vi "TCU Settings Dialog.vi"(8 "error in (no error)":errorcluster, 10 "Message Queues":T11, 11 "TCU Module State Cluster In":T1={"TCU Module Config"={"GUID"="", "Drop Coords"={"Horizontal"=0, "Vertical"=0}, "Process Name"="", "Queue Name"="", "Settings"={"Cycle Period"=500.0, "Setpoint Entry"=0.0, "Output Device"=enum."Default", "Huber Ministat 230 Settings"={"VISA resource name"="", "Simulated?"=TRUE}, "Lauda Settings"={"VISA resource name"="", "Simulated?"=FALSE, "Pump Power"=2}, "Julabo FP-50 Settings"={"VISA resource name"="", "Simulated?"=FALSE, "Pump Power"=2}, "Internal Control?"=FALSE, "Huber Unistat 410 Settings"={"VISA resource name"="", "Address"=0, "Simulated?"=FALSE}}, "Load Count"=0, "Power Level Changed"=FALSE}, "State"=enum."Idle", "Start Time"=timestamp(0 s since 1904-01-01), "Current Time"=timestamp(0 s since 1904-01-01), "First Iteration"=FALSE, "Data"={"TCU Temp"=0.0}, "Process Name"="", "TCU On?"=FALSE, "Power Level Changed"=FALSE} {"TCU Module Config"."Settings"."Huber Unistat 410 Settings"."Address" min=0 max=99 format="%02.0f"; "TCU Module Config"."Settings"."Julabo FP-50 Settings"."Pump Power" min=0 max=8 step=1; "TCU Module Config"."Settings"."Lauda Settings"."Pump Power" min=0 max=8 step=1}) -> (0 "error out":errorcluster, 1 "Cancelled?":bool=TRUE, 2 "UI Refresh Needed?":bool, 3 "TCU Module Config Out":T2={"GUID"="", "Drop Coords"={"Horizontal"=0, "Vertical"=0}, "Process Name"="", "Queue Name"="", "Settings"={"Cycle Period"=0.0, "Setpoint Entry"=0.0, "Output Device"=enum."Default", "Huber Ministat 230 Settings"={"VISA resource name"="", "Simulated?"=FALSE}, "Lauda Settings"={"VISA resource name"="", "Simulated?"=FALSE, "Pump Power"=2}, "Julabo FP-50 Settings"={"VISA resource name"="", "Simulated?"=FALSE, "Pump Power"=2}, "Internal Control?"=FALSE, "Huber Unistat 410 Settings"={"VISA resource name"="", "Address"=0, "Simulated?"=FALSE}}, "Load Count"=0, "Power Level Changed"=FALSE} {"Settings"."Huber Unistat 410 Settings"."Address" min=0 max=99 format="%02.0f"; "Settings"."Julabo FP-50 Settings"."Pump Power" min=0 max=8 step=1; "Settings"."Lauda Settings"."Pump Power" min=0 max=8 step=1})   [LabVIEW 2018, in "TCU Module.lvlib"]
doc: "Dialog for selecting user specified settings."
uses:
  TCU Module.lvlib
  Ismatec ISM 831C/Controls/Ismatech Settings Cluster.ctl
  Masterflex 7550-30/Controls/Settings Cluster.ctl
  VICI M50/VICI Settings.ctl
  Measure Instrument/Output Devices.ctl
  Huber TCU/Huber Settings.ctl
  Julabo Type 1 TCU/Julabo Type 1 TCU Folder/Julabo FP-50 Settings.ctl
  Lauda Integral XT-150 TCU/Lauda Settings.ctl
  Huber Unistat 410 TCU/Huber Unistat 410 RS485 Settings.ctl
  All Message Queues.ctl
  support/Message Queue/Message Cluster.ctl
  TCU Module Config Cluster.ctl
  <vilib>/Utility/miscctls.llb/LVPoint32TypeDef.ctl
  TCU Module Settings Cluster.ctl
  TCU Module State Cluster.ctl
  Measure Instrument/State Enum.ctl
  support/Message Queue/Enqueue Message (Single).vi
  <vilib>/Utility/xml.llb/Write to XML File(string).vi
  Settings/Settings.lvlib
  support/Support Library.lvlib
  support/Message Queue/Message Queue.lvlib
  Huber TCU/Huber Ministat 230 TCU.lvlib
  Lauda Integral XT-150 TCU/Lauda TCU.lvlib
  Julabo Type 1 TCU/Julabo Type 1 TCU Folder/Julabo Type FP-50 TCU.lvlib
  Huber Unistat 410 TCU/Huber Unistat 410 TCU.lvlib
  Ismatec ISM 831C/Ismatec ISM 831C.lvlib
  Masterflex 7550-30/Masterflex 7550-30.lvlib
  Measure Instrument/Feed Module Engine.lvlib
panel:
  in  "Module Name":string
  in  "TCU Settings":T15={"TCU Configuration"={"Cycle Period"=500.0, "Ismatech"={"VISA resource name"="", "Simulated?"=FALSE, "Pump Number"=1.0, "Reverse?"=FALSE}, "Masterflex"={"VISA resource name"="", "Simulated?"=FALSE, "Pump Number"=1.0, "Reverse?"=FALSE}, "Setpoint Entry"=0.0, "VICI Settings"={"VISA resource name"="", "Simulated?"=FALSE, "Pump Number"=0.0, "Reverse?"=FALSE}, "Output Device"=enum."Default", "Huber Ministat 230 Settings"={"VISA resource name"="", "Simulated?"=FALSE}, "Julabo Type 1 Settings"={"VISA resource name"="", "Simulated?"=FALSE, "Pump Power"=2}, "Lauda Settings"={"VISA resource name"="", "Simulated?"=FALSE, "Pump Power"=2}, "Control"=enum."Internal", "Huber Unistat 410 Settings"={"VISA resource name"="", "Address"=0, "Simulated?"=FALSE}}, "Stop"=FALSE, "Start"=FALSE} {"TCU Configuration"."Huber Unistat 410 Settings"."Address" min=0 max=99 format="%02.0f"; "TCU Configuration"."Lauda Settings"."Pump Power" min=0 max=8 step=1; "TCU Configuration"."Julabo Type 1 Settings"."Pump Power" min=0 max=8 step=1; "TCU Configuration"."VICI Settings"."Pump Number" min=1.0 max=20.0 step=1.0; "TCU Configuration"."Ismatech"."Pump Number" min=1.0 max=20.0 step=1.0; "TCU Configuration"."Masterflex"."Pump Number" min=1.0 max=20.0 step=1.0}
  in  "Cancel Button":bool
  in  "OK Button":bool
  # "Non visible portion of dialog (needed for connector pane)."
  # "Output Instruments"
  # "Output Instruments"
  # "Output Instruments"
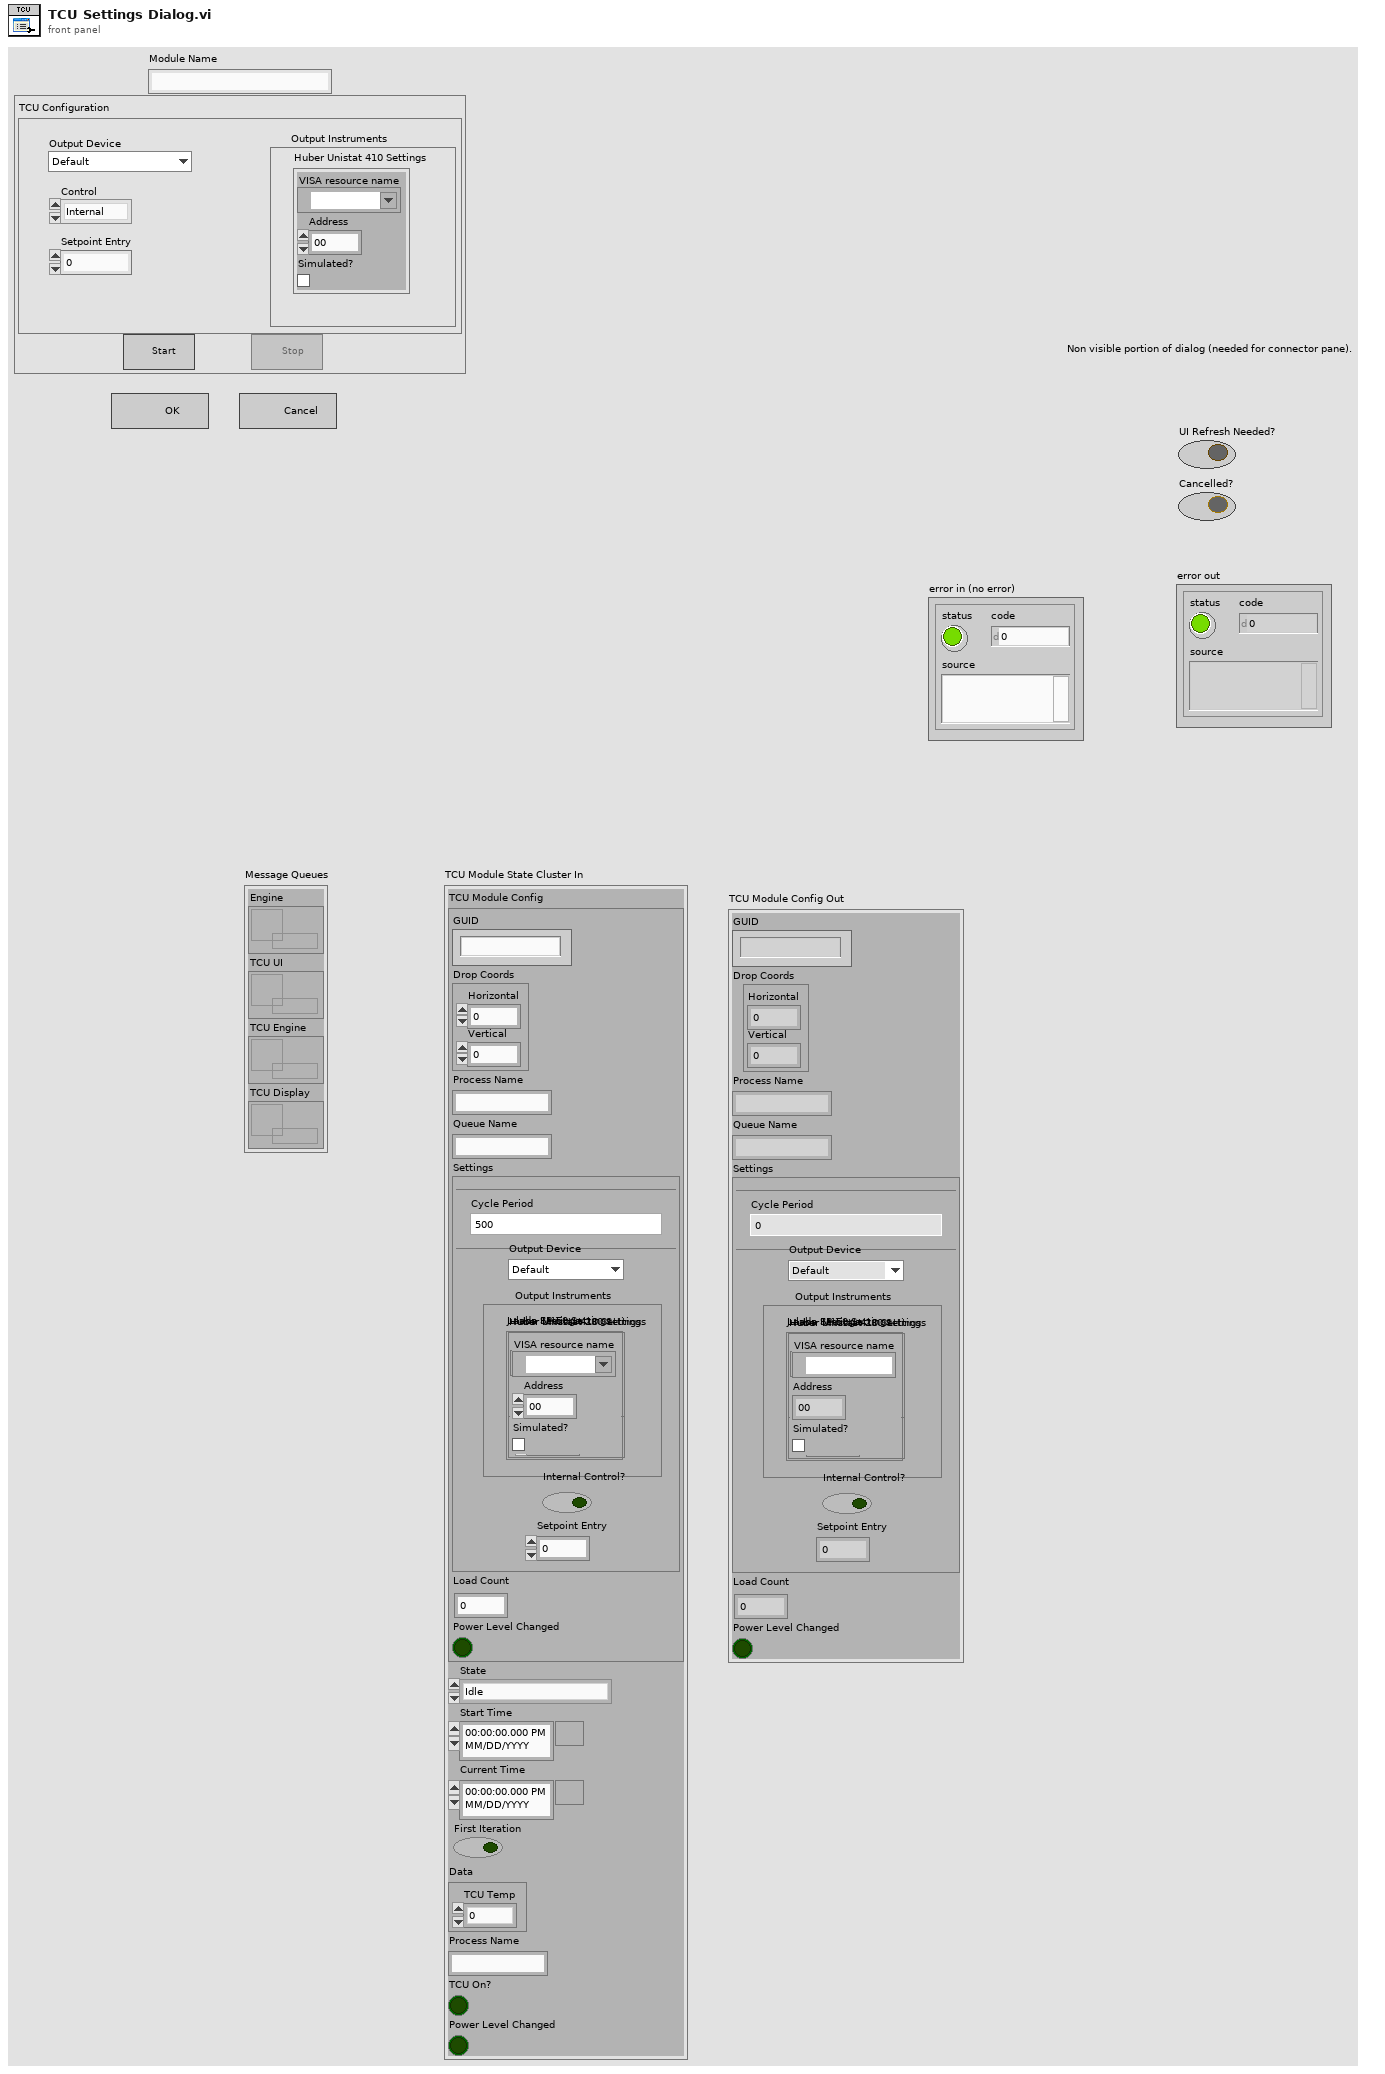
[diagram p1: front panel]
types:
  T1 = typedef "TCU Module.lvlib/TCU Module State Cluster.ctl" = cluster{"TCU Module Config":T2, "State":T10, "Start Time":timestamp, "Current Time":timestamp, "First Iteration":bool, "Data":cluster{"TCU Temp":dbl}, "Process Name":string, "TCU On?":bool, "Power Level Changed":bool}
  T2 = typedef "TCU Module.lvlib/TCU Module Config Cluster.ctl" = cluster{"GUID":string, "Drop Coords":T3, "Process Name":string, "Queue Name":string, "Settings":T4, "Load Count":i32, "Power Level Changed":bool}
  T3 = typedef "LVPoint32TypeDef.ctl" = cluster{"Horizontal":i32, "Vertical":i32}
  T4 = typedef "TCU Module.lvlib/TCU Module Settings Cluster.ctl" = cluster{"Cycle Period":dbl, "Setpoint Entry":dbl, "Output Device":T5, "Huber Ministat 230 Settings":T6, "Lauda Settings":T7, "Julabo FP-50 Settings":T8, "Internal Control?":bool, "Huber Unistat 410 Settings":T9}
  T5 = typedef "Output Devices.ctl" = enum16{"Default", "Huber Ministat 230", "Huber Unistat 410", "Lauda XT-150", "Julabo FP-50"}
  T6 = typedef "Huber Ministat 230 TCU.lvlib/Huber Settings.ctl" = cluster{"VISA resource name":refnum<visa-resource-name>, "Simulated?":bool}
  T7 = typedef "Lauda TCU.lvlib/Lauda Settings.ctl" = cluster{"VISA resource name":refnum<visa-resource-name>, "Simulated?":bool, "Pump Power":i32}
  T8 = typedef "Julabo Type FP-50 TCU.lvlib/Julabo FP-50 Settings.ctl" = cluster{"VISA resource name":refnum<visa-resource-name>, "Simulated?":bool, "Pump Power":i32}
  T9 = typedef "Huber Unistat 410 TCU.lvlib/Huber Unistat 410 RS485 Settings.ctl" = cluster{"VISA resource name":refnum<visa-resource-name>, "Address":i8, "Simulated?":bool}
  T10 = typedef "Feed Module.lvlib/Feed Module Engine.lvlib/State Enum.ctl" = enum16{"Measuring", "Idle", "Paused"}
  T11 = typedef "TCU Module.lvlib/All Message Queues.ctl" = cluster{"Engine":refnum<queue>, "TCU UI":refnum<queue>, "TCU Engine":refnum<queue>, "TCU Display":refnum<queue>}
  T12 = typedef "Ismatec ISM 831C.lvlib/Ismatech Settings Cluster.ctl" = cluster{"VISA resource name":refnum<visa-resource-name>, "Simulated?":bool, "Pump Number":dbl, "Reverse?":bool}
  T13 = typedef "Masterflex 7550-30.lvlib/Settings Cluster.ctl" = cluster{"VISA resource name":refnum<visa-resource-name>, "Simulated?":bool, "Pump Number":dbl, "Reverse?":bool}
  T14 = typedef "VICI Settings.ctl" = cluster{"VISA resource name":refnum<visa-resource-name>, "Simulated?":bool, "Pump Number":dbl, "Reverse?":bool}
  T15 = cluster{"TCU Configuration":cluster{"Cycle Period":dbl, "Ismatech":T12, "Masterflex":T13, "Setpoint Entry":dbl, "VICI Settings":T14, "Output Device":T5, "Huber Ministat 230 Settings":T6, "Julabo Type 1 Settings":T8, "Lauda Settings":T7, "Control":enum16{"Internal", "External"}, "Huber Unistat 410 Settings":T9}, "Stop":bool, "Start":bool}
  T16 = enum8{"Enabled", "Disabled", "Disabled and Grayed Out"}
  T17 = cluster{"Cycle Period":dbl, "Ismatech":T12, "Masterflex":T13, "Setpoint Entry":dbl, "VICI Settings":T14, "Output Device":T5, "Huber Ministat 230 Settings":T6, "Julabo Type 1 Settings":T8, "Lauda Settings":T7, "Control":enum16{"Internal", "External"}, "Huber Unistat 410 Settings":T9}
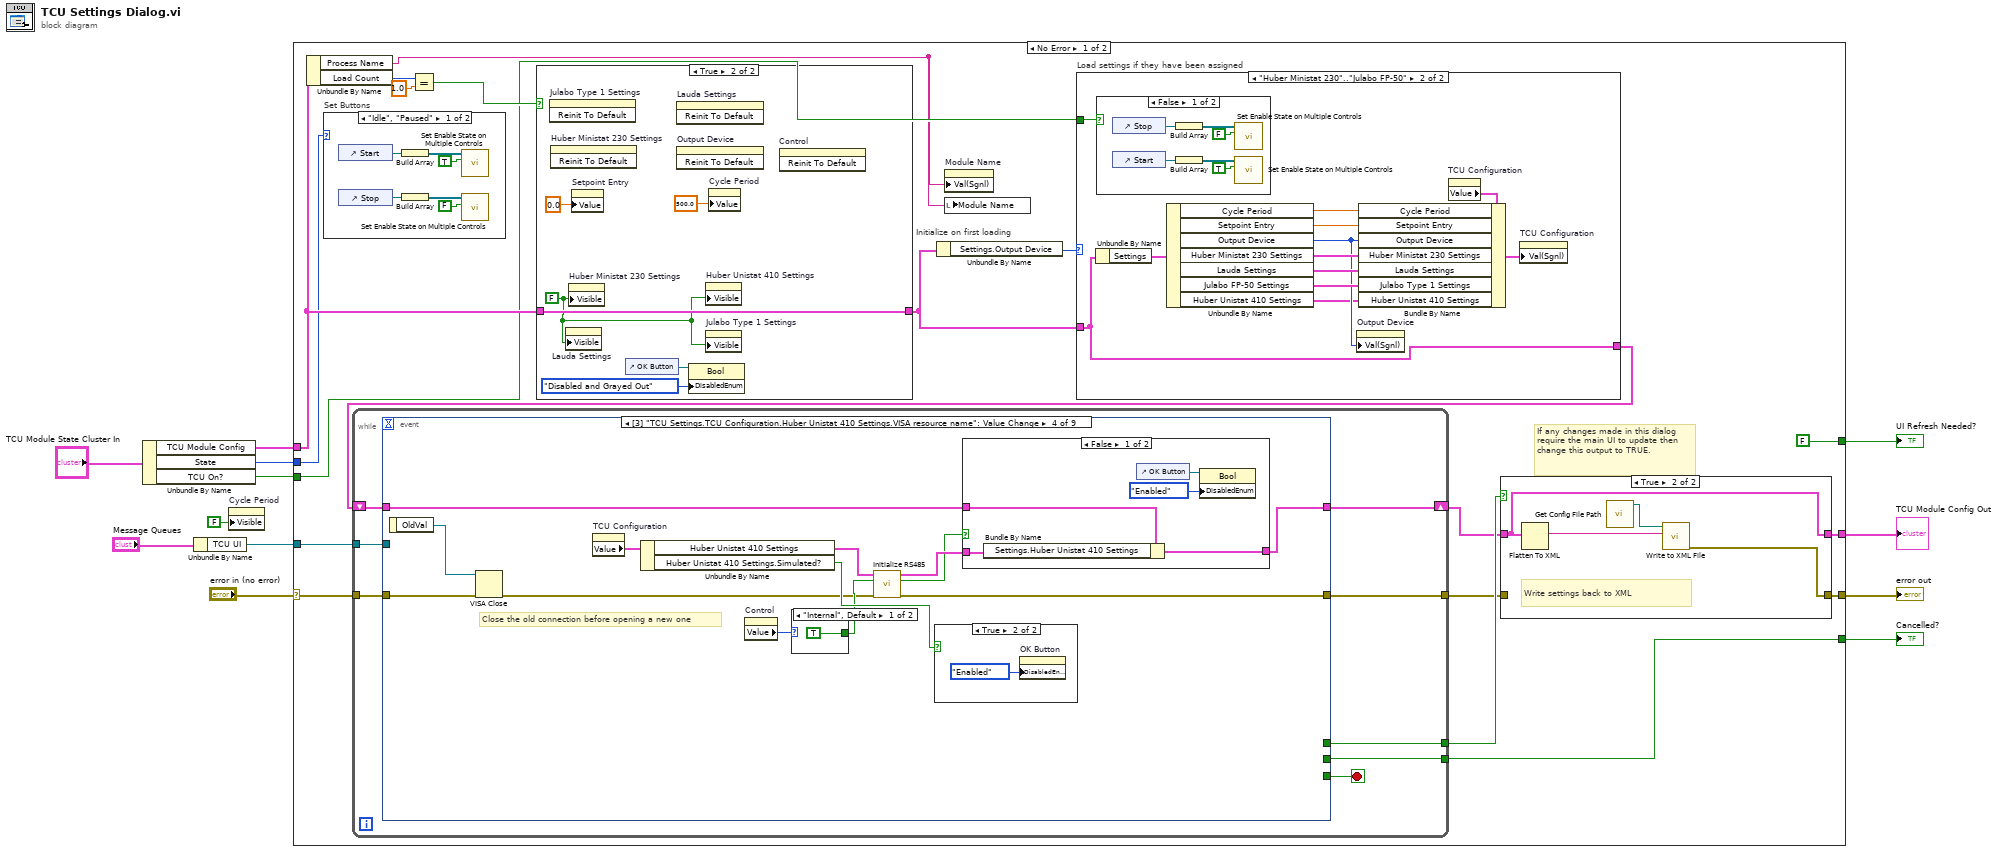
[diagram p0: block diagram]
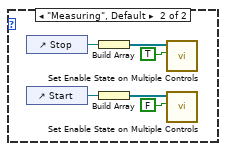
[diagram p2: hidden frame]
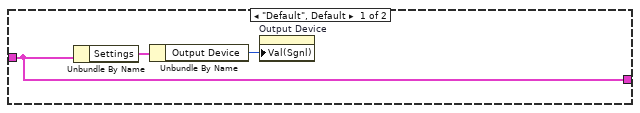
[diagram p3: hidden frame]
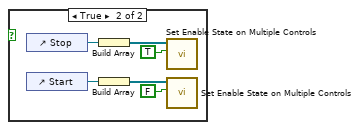
[diagram p4: hidden frame]
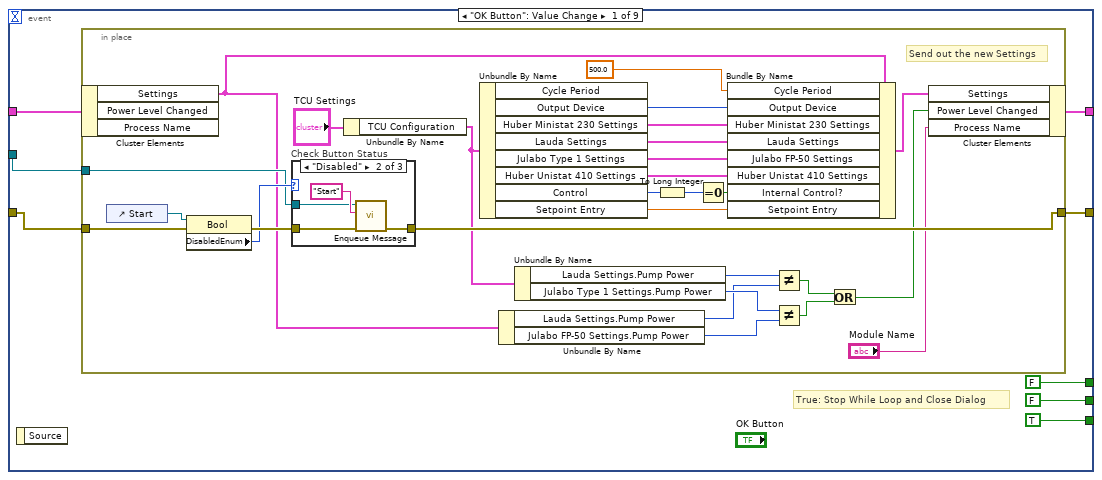
[diagram p6: hidden frame]
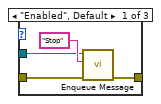
[diagram p7: hidden frame]
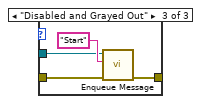
[diagram p8: hidden frame]
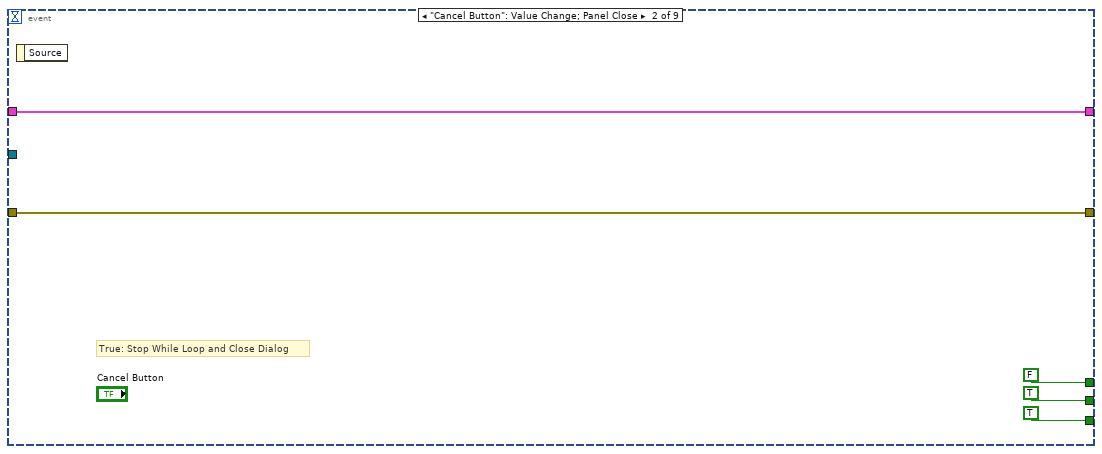
[diagram p9: hidden frame]
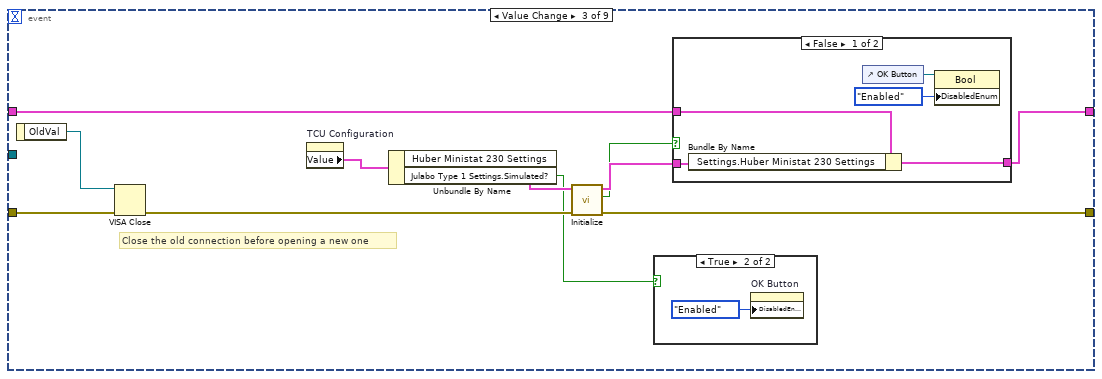
[diagram p10: hidden frame]
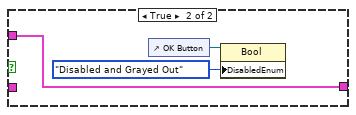
[diagram p12: hidden frame]
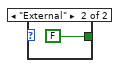
[diagram p14: hidden frame]
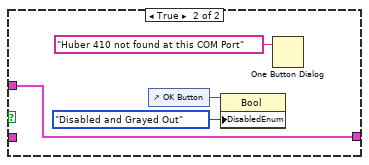
[diagram p15: hidden frame]
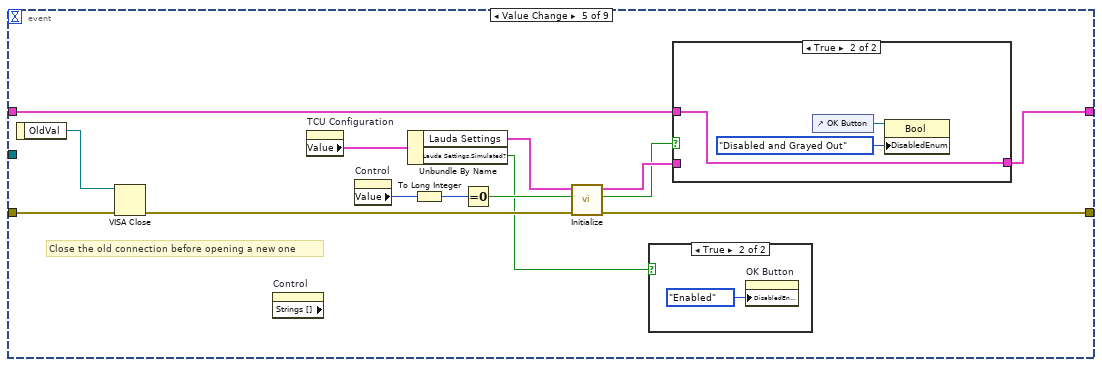
[diagram p16: hidden frame]
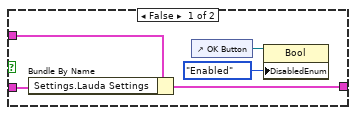
[diagram p18: hidden frame]
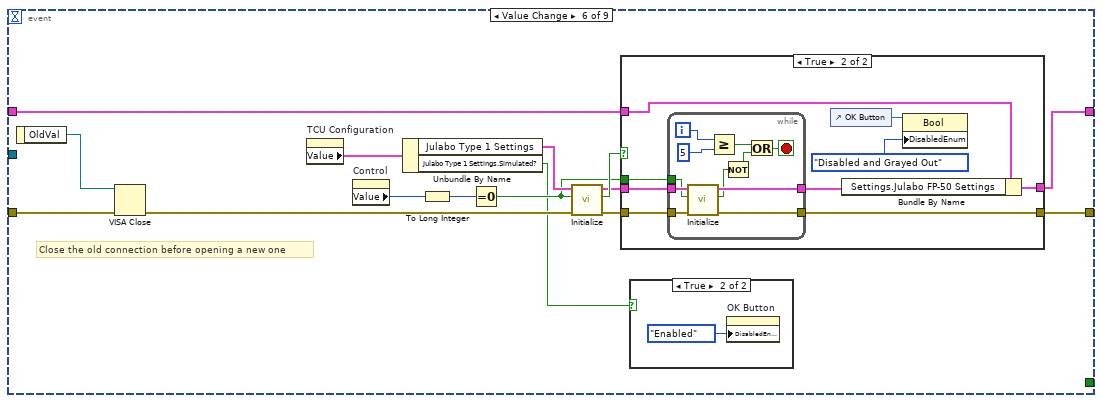
[diagram p19: hidden frame]
diagram:
  n1 = Unbundle By Name("TCU Module State Cluster In") -> ("TCU Module Config"=w4:T2, "State"=w3:T10, "TCU On?"=w1:bool)
  n2 = Unbundle By Name("Message Queues") -> ("TCU UI"=w9:refnum<queue>)
  n3 = property on="Cycle Period" class="DigNum (strict)"("Visible"=FALSE) -> ()  [unwired: 2 in, 2 out]
  n4 = case shown="No Error" "error in (no error)" {
    selector: "error in (no error)" -> [w18 w301]
    tunnel: [w21 w301] -> w12
    tunnel: w4 -> [w17 w299]
    tunnel: [w25 w299] -> w6
    tunnel: [FALSE ("UI Refresh Needed?") _] -> w11
    tunnel: [w28 TRUE ("UI Refresh Needed?")] -> w10
    tunnel: w9 -> [w19 _]
    tunnel: w3 -> [w15 _]
    tunnel: w1 -> [w14 _]
    frame No Error {
      # "If any changes made in this dialog require the main UI to update then change this output to TRUE."
      n5 = Unbundle By Name(w17) -> ("Process Name"=w13:string, "Load Count"=w30:i32)
      n6 = case "Set Buttons" shown="\"Idle\", \"Paused\"" w15 {
        frame "Idle", "Paused" {
          n7 = control-ref of="Start"() -> (w32:refnum<vi>)
          n8 = control-ref of="Stop"() -> (w34:refnum<vi>)
          n9 = Build Array(w32) -> (w36:refnum<vi>[])
          n10 = Build Array(w34) -> (w33:refnum<vi>[])
          n11 = call "Set Enable State on Multiple Controls.vi"("Enable?"=TRUE, "Controls"=w36) -> ()  [unwired: 10 in]
          n12 = call "Set Enable State on Multiple Controls.vi"("Enable?"=FALSE, "Controls"=w33) -> ()  [unwired: 10 in]
        }
        frame "Measuring", Default {
          n13 = control-ref of="Stop"() -> (w38:refnum<vi>)
          n14 = control-ref of="Start"() -> (w39:refnum<vi>)
          n15 = Build Array(w38) -> (w42:refnum<vi>[])
          n16 = Build Array(w39) -> (w40:refnum<vi>[])
          n17 = call "Set Enable State on Multiple Controls.vi"("Enable?"=TRUE, "Controls"=w42) -> ()  [unwired: 10 in]
          n18 = call "Set Enable State on Multiple Controls.vi"("Enable?"=FALSE, "Controls"=w40) -> ()  [unwired: 10 in]
        }
      }
      n19 = Equal?(x=w30, y=1.0) -> (x = y?=w24:bool)
      n20 = case "Initialize on first loading" shown="True" w24 {
        tunnel: w17 -> [w71 w77]
        tunnel: [w71 w77] -> w26
        frame False {
        }
        frame True {
          w72 = FALSE ("Visible")
          n21 = invoke on="Julabo Type 1 Settings" class="Clust (strict)" method="Reinit To Default"() -> ()  [unwired: 3 in, 3 out]
          n22 = invoke on="Huber Ministat 230 Settings" class="Clust (strict)" method="Reinit To Default"() -> ()  [unwired: 3 in, 3 out]
          n23 = property on="Lauda Settings" class="Clust (strict)"("Visible"=w72) -> ()  [unwired: 2 in, 2 out]
          n24 = property on="Huber Ministat 230 Settings" class="Clust (strict)"("Visible"=w72) -> ()  [unwired: 2 in, 2 out]
          n25 = property on="Setpoint Entry" class="DigNum (strict)"("Value"=0.0) -> ()  [unwired: 2 in, 2 out]
          n26 = control-ref of="OK Button"() -> (w74:refnum<vi>)
          n27 = invoke on="Lauda Settings" class="Clust (strict)" method="Reinit To Default"() -> ()  [unwired: 3 in, 3 out]
          n28 = invoke on="Output Device" class="Enum (strict)" method="Reinit To Default"() -> ()  [unwired: 3 in, 3 out]
          n29 = property class="Bool"(reference=w74, "DisabledEnum"=T16."Disabled and Grayed Out" ("Disabled")) -> ()  [unwired: 1 in, 2 out]
          n30 = property on="Huber Unistat 410 Settings" class="Clust (strict)"("Visible"=w72) -> ()  [unwired: 2 in, 2 out]
          n31 = property on="Julabo Type 1 Settings" class="Clust (strict)"("Visible"=w72) -> ()  [unwired: 2 in, 2 out]
          n32 = property on="Cycle Period" class="DigNum (strict)"("Value"=500.0) -> ()  [unwired: 2 in, 2 out]
          n33 = invoke on="Control" class="Enum (strict)" method="Reinit To Default"() -> ()  [unwired: 3 in, 3 out]
        }
      }
      n34 = Unbundle By Name(w26) -> ("Settings.Output Device"=w27:T5)
      n35 = local write "Module Name"(w13) -> ()
      n36 = property on="Module Name" class="Str"("Val(Sgnl)"=w13) -> ()  [unwired: 2 in, 2 out]
      n37 = case "Load settings if they have been assigned" shown="\"Huber Ministat 230\"..\"Julabo FP-50\"" w27 {
        tunnel: w26 -> [w44 w48]
        tunnel: [w44 w48] -> w16
        tunnel: w14 -> [_ w51]
        frame "Default", Default {
          n38 = Unbundle By Name(w44) -> ("Settings"=w46:T4)
          n39 = Unbundle By Name(w46) -> ("Output Device"=w45:T5)
          n40 = property on="Output Device" class="Enum (strict)"("Val(Sgnl)"=w45) -> ()  [unwired: 2 in, 2 out]
        }
        frame "Huber Ministat 230".."Julabo FP-50" {
          n41 = Unbundle By Name(w48) -> ("Settings"=w56:T4)
          n42 = case shown="False" w51 {
            frame False {
              n43 = control-ref of="Stop"() -> (w61:refnum<vi>)
              n44 = control-ref of="Start"() -> (w62:refnum<vi>)
              n45 = Build Array(w61) -> (w63:refnum<vi>[])
              n46 = Build Array(w62) -> (w64:refnum<vi>[])
              n47 = call "Set Enable State on Multiple Controls.vi"("Enable?"=FALSE, "Controls"=w63) -> ()  [unwired: 10 in]
              n48 = call "Set Enable State on Multiple Controls.vi"("Enable?"=TRUE, "Controls"=w64) -> ()  [unwired: 10 in]
            }
            frame True {
              n49 = control-ref of="Stop"() -> (w67:refnum<vi>)
              n50 = control-ref of="Start"() -> (w68:refnum<vi>)
              n51 = Build Array(w67) -> (w69:refnum<vi>[])
              n52 = Build Array(w68) -> (w70:refnum<vi>[])
              n53 = call "Set Enable State on Multiple Controls.vi"("Enable?"=TRUE, "Controls"=w69) -> ()  [unwired: 10 in]
              n54 = call "Set Enable State on Multiple Controls.vi"("Enable?"=FALSE, "Controls"=w70) -> ()  [unwired: 10 in]
            }
          }
          n55 = Unbundle By Name(w56) -> ("Cycle Period"=w58:dbl, "Setpoint Entry"=w54:dbl, "Output Device"=w49:T5, "Huber Ministat 230 Settings"=w55:T6, "Lauda Settings"=w53:T7, "Julabo FP-50 Settings"=w52:T8, "Huber Unistat 410 Settings"=w47:T9)
          n56 = property on="Output Device" class="Enum (strict)"("Val(Sgnl)"=w49) -> ()  [unwired: 2 in, 2 out]
          n57 = property on="TCU Configuration" class="Clust (strict)"() -> ("Value"=w50:T17)  [unwired: 2 in, 2 out]
          n58 = Bundle By Name(cluster=w50, "Cycle Period"=w58, "Setpoint Entry"=w54, "Output Device"=w49, "Huber Ministat 230 Settings"=w55, "Lauda Settings"=w53, "Julabo Type 1 Settings"=w52, "Huber Unistat 410 Settings"=w47) -> (w57:T17)
          n59 = property on="TCU Configuration" class="Clust (strict)"("Val(Sgnl)"=w57) -> ()  [unwired: 2 in, 2 out]
        }
      }
      n60 = while {
        tunnel: [w85] -> w23
        tunnel: [w83] -> w28
        tunnel: [w81] -> w20
        tunnel: w19 -> [w80]
        tunnel: w18 -> [w79]
        shift-right: [w82] -> w22
        shift-left: w16 -> [w78]
        stop <- w84 stop-if-true
        n61 = event shown="[3] \"TCU Settings.TCU Configuration.Huber Unistat 410 Settings.VISA resource name\": Value Change" {
          selector: _ -> [_ _ _ _ _ _ _ _ _]
          dyn-events: _ -> [_ _ _ _ _ _ _ _ _]
          timeout: _ -> [_ _ _ _ _ _ _ _ _]
          tunnel: [FALSE ("UI Refresh Needed?") FALSE ("UI Refresh Needed?") _ _ _ _ _ _ _] -> w85
          tunnel: [TRUE TRUE _ _ _ _ _ _ _] -> w84
          tunnel: [FALSE ("UI Refresh Needed?") TRUE ("UI Refresh Needed?") _ _ _ _ _ _ _] -> w83
          tunnel: w78 -> [w87 w135 w147 w169 w195 w212 w250 w278 w286]
          tunnel: [w86 w135 w146 w168 w194 w211 w249 w278 w286] -> w82
          tunnel: [w90 w134 w143 w159 w189 w209 _ w277 w285] -> w81
          tunnel: w80 -> [w89 _ _ _ _ _ _ _ _]
          tunnel: w79 -> [w88 w134 w145 w167 w193 w219 _ w277 w285]
          event "OK Button": Value Change {
            # "True: Stop While Loop and Close Dialog"
            n62 = event-data() -> ()  [unwired: 1 in, 1 out]
            n63 = in-place {
              in-place-border: [w117] -> w90
              in-place-border: w89 -> [w116]
              in-place-border: w88 -> [w115]
              # "Send out the new Settings"
              n64 = in-place-cluster #1(w87) -> ("Settings"=w95:T4)  [unwired: 2 out]
              n65 = control-ref of="Start"() -> (w120:refnum<vi>)
              n66 = property class="Bool"(reference=w120, error in=w115) -> (error out=w121:errorcluster, "DisabledEnum"=w118:T16)  [unwired: 1 out]
              n67 = case "Check Button Status" shown="\"Disabled\"" w118 {
                tunnel: w121 -> [w123 w128 w132]
                tunnel: [w125 w127 w131] -> w117
                tunnel: w116 -> [w122 w126 w130]
                frame "Enabled", Default {
                  n68 = call-poly "Enqueue Message.vi"("error in (no error)"=w123, "Message"="Stop", "Message Queue"=w122) -> ("error out"=w125:errorcluster)  [unwired: 7 in, 1 out]
                }
                frame "Disabled" {
                  n69 = call-poly "Enqueue Message.vi"("error in (no error)"=w128, "Message"="Start", "Message Queue"=w126) -> ("error out"=w127:errorcluster)  [unwired: 7 in, 1 out]
                }
                frame "Disabled and Grayed Out" {
                  n70 = call-poly "Enqueue Message.vi"("error in (no error)"=w132, "Message"="Start", "Message Queue"=w130) -> ("error out"=w131:errorcluster)  [unwired: 7 in, 1 out]
                }
              }
              n71 = Unbundle By Name("TCU Settings") -> ("TCU Configuration"=w105:T17)
              n72 = Unbundle By Name(w105) -> ("Output Device"=w114:T5, "Huber Ministat 230 Settings"=w109:T6, "Lauda Settings"=w110:T7, "Julabo Type 1 Settings"=w113:T8, "Huber Unistat 410 Settings"=w94:T9, "Control"=w108:enum16{"Internal", "External"}, "Setpoint Entry"=w111:dbl)  [unwired: 1 out]
              n73 = Unbundle By Name(w95) -> ("Lauda Settings.Pump Power"=w97:i32, "Julabo FP-50 Settings.Pump Power"=w96:i32)
              n74 = Unbundle By Name(w105) -> ("Lauda Settings.Pump Power"=w104:i32, "Julabo Type 1 Settings.Pump Power"=w101:i32)
              n75 = To Long Integer(number=w108) -> (32bit integer=w107:i32)
              n76 = Equal To 0?(x=w107) -> (x = 0?=w106:bool)
              n77 = Bundle By Name(cluster=w95, "Cycle Period"=500.0, "Output Device"=w114, "Huber Ministat 230 Settings"=w109, "Lauda Settings"=w110, "Julabo FP-50 Settings"=w113, "Huber Unistat 410 Settings"=w94, "Internal Control?"=w106, "Setpoint Entry"=w111) -> (w100:T4)
              n78 = Not Equal?(x=w104, y=w97) -> (x != y?=w103:bool)
              n79 = Not Equal?(x=w101, y=w96) -> (x != y?=w102:bool)
              n80 = Or(x=w103, y=w102) -> (x .or. y?=w99:bool)
              n81 = in-place-cluster #1("Settings"=w100, "Power Level Changed"=w99, "Process Name"="Module Name") -> (w86:T2)
            }
          }
          event "Cancel Button": Value Change; Panel Close {
            # "True: Stop While Loop and Close Dialog"
            n82 = event-data() -> ()  [unwired: 1 in, 1 out]
          }
          event Value Change {
            # "Close the old connection before opening a new one"
            n83 = event-data() -> ("OldVal"=w148:refnum<visa-resource-name>)  [unwired: 1 in]
            n84 = VISA Close(VISA resource name=w148, error in (no error)=w145) -> (error out=w144:errorcluster)
            n85 = property on="TCU Configuration" class="Clust (strict)"() -> ("Value"=w149:T17)  [unwired: 2 in, 2 out]
            n86 = Unbundle By Name(w149) -> ("Huber Ministat 230 Settings"=w142:T6, "Julabo Type 1 Settings.Simulated?"=w139:bool)
            n87 = call "Initialize.vi"("error in (no error)"=w144, "Huber Settings"=w142) -> ("error out"=w143:errorcluster, "Connection Error"=w140:bool, "Huber Settings"=w141:T6)  [unwired: 7 in]
            n88 = case shown="True" w139 {
              frame False {
              }
              frame True {
                n89 = property on="OK Button" class="Bool"("DisabledEnum"=T16."Enabled" ("Disabled")) -> ()  [unwired: 2 in, 2 out]
              }
            }
            n90 = case shown="False" w140 {
              tunnel: w141 -> [w155 _]
              tunnel: w147 -> [w151 w158]
              tunnel: [w154 w158] -> w146
              frame False {
                n91 = Bundle By Name(cluster=w151, "Settings.Huber Ministat 230 Settings"=w155) -> (w154:T2)
                n92 = control-ref of="OK Button"() -> (w152:refnum<vi>)
                n93 = property class="Bool"(reference=w152, "DisabledEnum"=T16."Enabled" ("Disabled")) -> ()  [unwired: 1 in, 2 out]
              }
              frame True {
                n94 = control-ref of="OK Button"() -> (w156:refnum<vi>)
                n95 = property class="Bool"(reference=w156, "DisabledEnum"=T16."Disabled and Grayed Out" ("Disabled")) -> ()  [unwired: 1 in, 2 out]
              }
            }
          }
          event Value Change {
            # "Close the old connection before opening a new one"
            n96 = event-data() -> ("OldVal"=w170:refnum<visa-resource-name>)  [unwired: 1 in]
            n97 = VISA Close(VISA resource name=w170, error in (no error)=w167) -> (error out=w162:errorcluster)
            n98 = property on="TCU Configuration" class="Clust (strict)"() -> ("Value"=w171:T17)  [unwired: 2 in, 2 out]
            n99 = Unbundle By Name(w171) -> ("Huber Unistat 410 Settings"=w164:T9, "Huber Unistat 410 Settings.Simulated?"=w165:bool)
            n100 = property on="Control" class="Enum (strict)"() -> ("Value"=w166:enum16{"Internal", "External"})  [unwired: 2 in, 2 out]
            n101 = case shown="\"Internal\", Default" w166 {
              tunnel: [TRUE FALSE] -> w163
              frame "Internal", Default {
              }
              frame "External" {
              }
            }
            n102 = call "Initialize RS485.vi"("error in (no error)"=w162, "Internal?"=w163, "Huber Unistat 410 Settings"=w164) -> ("error out"=w159:errorcluster, "Connection Error"=w160:bool, "Huber Unistat 410 Settings 2"=w161:T9)  [unwired: 6 in]
            n103 = case shown="True" w165 {
              frame False {
              }
              frame True {
                n104 = property on="OK Button" class="Bool"("DisabledEnum"=T16."Enabled" ("Disabled")) -> ()  [unwired: 2 in, 2 out]
              }
            }
            n105 = case shown="False" w160 {
              tunnel: w161 -> [w179 _]
              tunnel: w169 -> [w175 w183]
              tunnel: [w178 w183] -> w168
              frame False {
                n106 = Bundle By Name(cluster=w175, "Settings.Huber Unistat 410 Settings"=w179) -> (w178:T2)
                n107 = control-ref of="OK Button"() -> (w176:refnum<vi>)
                n108 = property class="Bool"(reference=w176, "DisabledEnum"=T16."Enabled" ("Disabled")) -> ()  [unwired: 1 in, 2 out]
              }
              frame True {
                n109 = control-ref of="OK Button"() -> (w181:refnum<vi>)
                n110 = property class="Bool"(reference=w181, "DisabledEnum"=T16."Disabled and Grayed Out" ("Disabled")) -> ()  [unwired: 1 in, 2 out]
                n111 = One Button Dialog(message="Huber 410 not found at this COM Port") -> ()  [unwired: 1 in, 1 out]
              }
            }
          }
          event Value Change {
            # "Close the old connection before opening a new one"
            n112 = event-data() -> ("OldVal"=w196:refnum<visa-resource-name>)  [unwired: 1 in]
            n113 = VISA Close(VISA resource name=w196, error in (no error)=w193) -> (error out=w192:errorcluster)
            n114 = property on="Control" class="Enum (strict)" props=["Strings []"]() -> ()  [unwired: 2 in, 3 out]
            n115 = property on="TCU Configuration" class="Clust (strict)"() -> ("Value"=w197:T17)  [unwired: 2 in, 2 out]
            n116 = property on="Control" class="Enum (strict)"() -> ("Value"=w185:enum16{"Internal", "External"})  [unwired: 2 in, 2 out]
            n117 = Unbundle By Name(w197) -> ("Lauda Settings"=w191:T7, "Lauda Settings.Simulated?"=w184:bool)
            n118 = To Long Integer(number=w185) -> (32bit integer=w186:i32)
            n119 = Equal To 0?(x=w186) -> (x = 0?=w188:bool)
            n120 = call "Initialize.vi"("error in (no error)"=w192, "Internal?"=w188, "Lauda Settings In"=w191) -> ("error out"=w189:errorcluster, "Connection Error"=w187:bool, "Lauda Settings Out"=w190:T7)  [unwired: 6 in]
            n121 = case shown="True" w184 {
              frame False {
              }
              frame True {
                n122 = property on="OK Button" class="Bool"("DisabledEnum"=T16."Enabled" ("Disabled")) -> ()  [unwired: 2 in, 2 out]
              }
            }
            n123 = case shown="True" w187 {
              tunnel: w190 -> [w203 _]
              tunnel: w195 -> [w199 w206]
              tunnel: [w202 w206] -> w194
              frame False {
                n124 = Bundle By Name(cluster=w199, "Settings.Lauda Settings"=w203) -> (w202:T2)
                n125 = control-ref of="OK Button"() -> (w200:refnum<vi>)
                n126 = property class="Bool"(reference=w200, "DisabledEnum"=T16."Enabled" ("Disabled")) -> ()  [unwired: 1 in, 2 out]
              }
              frame True {
                n127 = control-ref of="OK Button"() -> (w204:refnum<vi>)
                n128 = property class="Bool"(reference=w204, "DisabledEnum"=T16."Disabled and Grayed Out" ("Disabled")) -> ()  [unwired: 1 in, 2 out]
              }
            }
          }
          event Value Change {
            # "Close the old connection before opening a new one"
            n129 = event-data() -> ("OldVal"=w220:refnum<visa-resource-name>)  [unwired: 1 in]
            n130 = VISA Close(VISA resource name=w220, error in (no error)=w219) -> (error out=w218:errorcluster)
            n131 = property on="TCU Configuration" class="Clust (strict)"() -> ("Value"=w221:T17)  [unwired: 2 in, 2 out]
            n132 = property on="Control" class="Enum (strict)"() -> ("Value"=w215:enum16{"Internal", "External"})  [unwired: 2 in, 2 out]
            n133 = Unbundle By Name(w221) -> ("Julabo Type 1 Settings"=w217:T8, "Julabo Type 1 Settings.Simulated?"=w207:bool)
            n134 = To Long Integer(number=w215) -> (32bit integer=w216:i32)
            n135 = Equal To 0?(x=w216) -> (x = 0?=w208:bool)
            n136 = call "Initialize.vi"("error in (no error)"=w218, "Internal?"=w208, "Julabo FP-50 Settings"=w217) -> ("error out"=w210:errorcluster, "Connection Error"=w214:bool, "Julabo FP-50 Settings"=w213:T8)  [unwired: 6 in]
            n137 = case shown="True" w214 {
              tunnel: w213 -> [w226 w237]
              tunnel: w212 -> [w225 w234]
              tunnel: [w224 w235] -> w211
              tunnel: w210 -> [w223 w231]
              tunnel: [w223 w230] -> w209
              tunnel: w208 -> [_ w229]
              frame False {
                n138 = Bundle By Name(cluster=w225, "Settings.Julabo FP-50 Settings"=w226) -> (w224:T2)
                n139 = control-ref of="OK Button"() -> (w228:refnum<vi>)
                n140 = property class="Bool"(reference=w228, "DisabledEnum"=T16."Enabled" ("Disabled")) -> ()  [unwired: 1 in, 2 out]
              }
              frame True {
                n141 = while {
                  tunnel: w237 -> [w248]
                  tunnel: [w247] -> w236
                  tunnel: w231 -> [w242]
                  tunnel: [w241] -> w230
                  tunnel: w229 -> [w238]
                  i -> [w245]
                  stop <- w243 stop-if-true
                  n142 = call "Initialize.vi"("error in (no error)"=w242, "Internal?"=w238, "Julabo FP-50 Settings"=w248) -> ("error out"=w241:errorcluster, "Connection Error"=w246:bool, "Julabo FP-50 Settings"=w247:T8)  [unwired: 6 in]
                  n143 = Greater Or Equal?(x=w245, y=5) -> (x >= y?=w239:bool)
                  n144 = Not(x=w246) -> (.not. x?=w240:bool)
                  n145 = Or(x=w239, y=w240) -> (x .or. y?=w243:bool)
                }
                n146 = control-ref of="OK Button"() -> (w233:refnum<vi>)
                n147 = Bundle By Name(cluster=w234, "Settings.Julabo FP-50 Settings"=w236) -> (w235:T2)
                n148 = property class="Bool"(reference=w233, "DisabledEnum"=T16."Disabled and Grayed Out" ("Disabled")) -> ()  [unwired: 1 in, 2 out]
              }
            }
            n149 = case shown="True" w207 {
              frame False {
              }
              frame True {
                n150 = property on="OK Button" class="Bool"("DisabledEnum"=T16."Enabled" ("Disabled")) -> ()  [unwired: 2 in, 2 out]
              }
            }
          }
          event Value Change {
            n151 = event-data() -> ("NewVal"=w251:T5)  [unwired: 1 in]
            n152 = case "Selected Device" shown="\"Huber Unistat 410\"" w251 {
              tunnel: w250 -> [w256 w261 w262 w268 w273]
              tunnel: [w256 w261 w262 w268 w273] -> w249
              frame "Default", Default {
                n153 = property on="Huber Unistat 410 Settings" class="Clust (strict)"("Visible"=FALSE) -> ()  [unwired: 2 in, 2 out]
                n154 = property on="Julabo Type 1 Settings" class="Clust (strict)"("Visible"=FALSE) -> ()  [unwired: 2 in, 2 out]
                n155 = property on="Lauda Settings" class="Clust (strict)"("Visible"=FALSE) -> ()  [unwired: 2 in, 2 out]
                n156 = property on="Huber Ministat 230 Settings" class="Clust (strict)"("Visible"=FALSE) -> ()  [unwired: 2 in, 2 out]
              }
              frame "Huber Ministat 230" {
                n157 = property on="Huber Unistat 410 Settings" class="Clust (strict)"("Visible"=FALSE) -> ()  [unwired: 2 in, 2 out]
                n158 = property on="Julabo Type 1 Settings" class="Clust (strict)"("Visible"=FALSE) -> ()  [unwired: 2 in, 2 out]
                n159 = property on="Lauda Settings" class="Clust (strict)"("Visible"=FALSE) -> ()  [unwired: 2 in, 2 out]
                n160 = property on="Huber Ministat 230 Settings" class="Clust (strict)"("Visible"=TRUE) -> ()  [unwired: 2 in, 2 out]
              }
              frame "Huber Unistat 410" {
                n161 = property on="Huber Unistat 410 Settings" class="Clust (strict)"("Visible"=TRUE) -> ()  [unwired: 2 in, 2 out]
                n162 = property on="Julabo Type 1 Settings" class="Clust (strict)"("Visible"=FALSE) -> ()  [unwired: 2 in, 2 out]
                n163 = property on="Lauda Settings" class="Clust (strict)"("Visible"=FALSE) -> ()  [unwired: 2 in, 2 out]
                n164 = property on="Huber Ministat 230 Settings" class="Clust (strict)"("Visible"=FALSE) -> ()  [unwired: 2 in, 2 out]
              }
              frame "Lauda XT-150" {
                n165 = property on="Huber Unistat 410 Settings" class="Clust (strict)"("Visible"=FALSE) -> ()  [unwired: 2 in, 2 out]
                n166 = property on="Julabo Type 1 Settings" class="Clust (strict)"("Visible"=FALSE) -> ()  [unwired: 2 in, 2 out]
                n167 = property on="Lauda Settings" class="Clust (strict)"("Visible"=TRUE) -> ()  [unwired: 2 in, 2 out]
                n168 = property on="Huber Ministat 230 Settings" class="Clust (strict)"("Visible"=FALSE) -> ()  [unwired: 2 in, 2 out]
              }
              frame "Julabo FP-50" {
                n169 = property on="Huber Unistat 410 Settings" class="Clust (strict)"("Visible"=FALSE) -> ()  [unwired: 2 in, 2 out]
                n170 = property on="Julabo Type 1 Settings" class="Clust (strict)"("Visible"=TRUE) -> ()  [unwired: 2 in, 2 out]
                n171 = property on="Lauda Settings" class="Clust (strict)"("Visible"=FALSE) -> ()  [unwired: 2 in, 2 out]
                n172 = property on="Huber Ministat 230 Settings" class="Clust (strict)"("Visible"=FALSE) -> ()  [unwired: 2 in, 2 out]
              }
            }
          }
          event "TCU Settings.Start": Value Change {
            # "Enable Stop"
            # "Disable and Gray out Start"
            n173 = event-data() -> ()  [unwired: 1 in, 6 out]
            n174 = control-ref of="Start"() -> (w280:refnum<vi>)
            n175 = control-ref of="Stop"() -> (w279:refnum<vi>)
            n176 = Build Array(w280) -> (w282:refnum<vi>[])
            n177 = Build Array(w279) -> (w284:refnum<vi>[])
            n178 = call "Set Enable State on Multiple Controls.vi"("Enable?"=FALSE, "Controls"=w282) -> ()  [unwired: 10 in]
            n179 = call "Set Enable State on Multiple Controls.vi"("Enable?"=TRUE, "Controls"=w284) -> ()  [unwired: 10 in]
          }
          event "TCU Settings.Stop": Value Change {
            # "Enable Start"
            # "Disable and Gray out Stop"
            n180 = event-data() -> ()  [unwired: 1 in, 1 out]
            n181 = control-ref of="Stop"() -> (w287:refnum<vi>)
            n182 = control-ref of="Start"() -> (w288:refnum<vi>)
            n183 = Build Array(w287) -> (w290:refnum<vi>[])
            n184 = Build Array(w288) -> (w292:refnum<vi>[])
            n185 = call "Set Enable State on Multiple Controls.vi"("Enable?"=FALSE, "Controls"=w290) -> ()  [unwired: 10 in]
            n186 = call "Set Enable State on Multiple Controls.vi"("Enable?"=TRUE, "Controls"=w292) -> ()  [unwired: 10 in]
          }
        }
      }
      n187 = case shown="True" w23 {
        tunnel: w22 -> [w294 w295]
        tunnel: [w293 w296] -> w21
        tunnel: [w294 w295] -> w25
        tunnel: w20 -> [w293 _]
        frame False {
        }
        frame True {
          # "Write settings back to XML"
          n188 = Flatten To XML(anything=w295) -> (xml string=w297:string)
          n189 = call "Get Config File Path.vi"() -> ("XML File Path"=w298:path)  [unwired: 10 in, 1 out]
          n190 = call-poly <vilib>:"Write to XML File.vi"("XML Input"=w297, "XML File Path"=w298) -> ("error out"=w296:errorcluster)  [unwired: 7 in, 2 out]
        }
      }
    }
    frame Error {
    }
  }
  "UI Refresh Needed?" <- w11
  "error out" <- w12
  "Cancelled?" <- w10
  "TCU Module Config Out" <- w6
